vi "WidthEstimation.vi"(2 "maximum index":i32[](array[numeric]), 3 "maximium":dbl, 4 "2D Gaussian Data":dbl[][](array[numeric])) -> (0 "wy Estimated":dbl, 1 "wx Estimated":dbl)   [LabVIEW 2015]
panel:
  out "wx left":i32
  out "value wx left":dbl
  out "wx right":i32
  out "value wx right":dbl
  out "wy up":i32
  out "value wy up":dbl
  out "wy down":i32
  out "value wy down":dbl
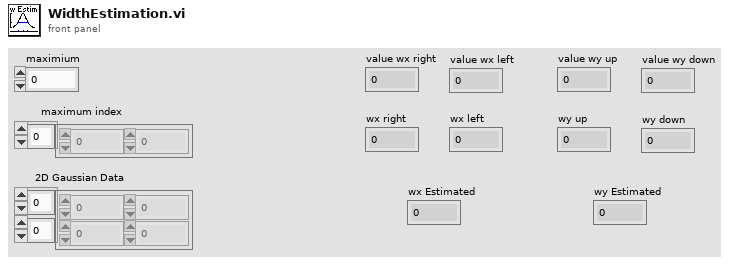
[diagram p1: front panel]
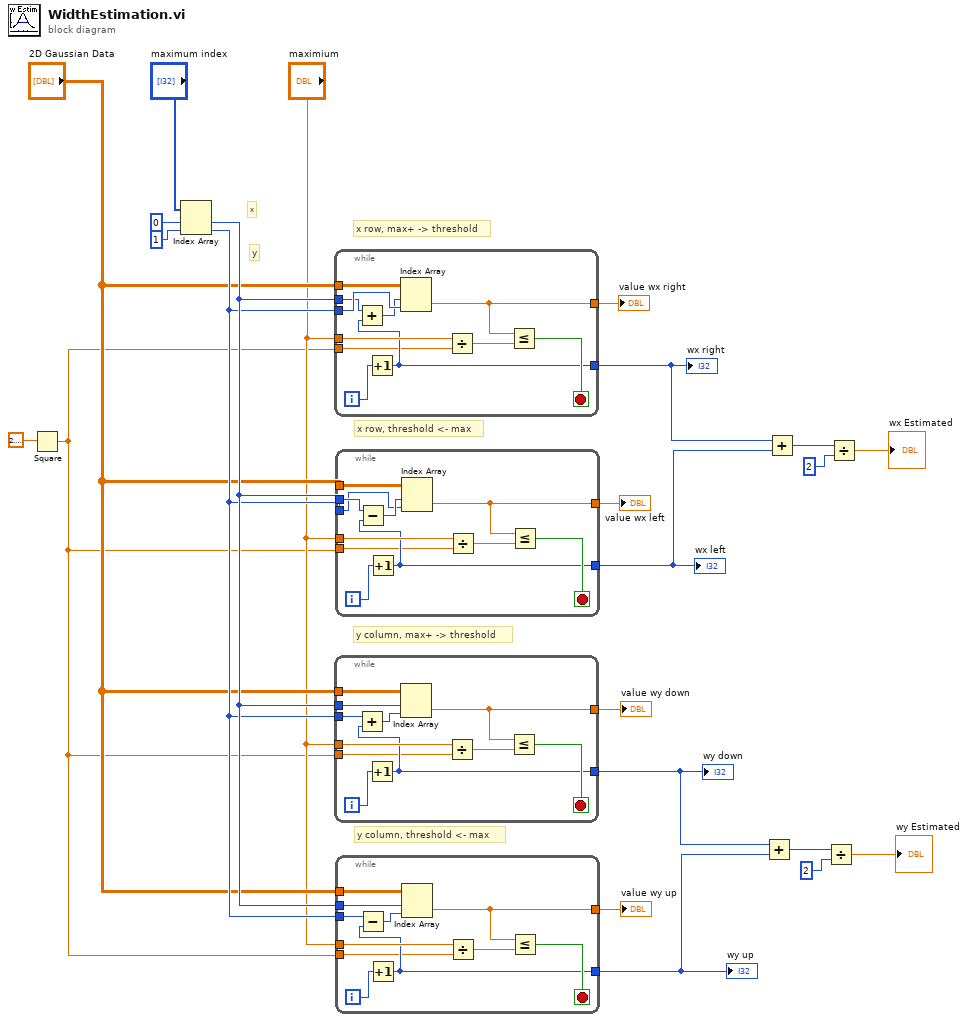
[diagram p0: block diagram]
diagram:
  # "x row, threshold <- max"
  # "x row, max+ -> threshold"
  # "y column, threshold <- max"
  # "y column, max+ -> threshold"
  # "y"
  # "x"
  n1 = Square(x=2.718281828459045) -> (x^2=w1:dbl)
  n2 = Index Array(array="maximum index", index #1=0 ("index"), index #2=1 ("index")) -> (element #1=w13:i32, element #2=w12:i32)
  n3 = while {
    tunnel: "2D Gaussian Data" -> [w34]
    tunnel: w13 -> [w26]
    tunnel: w12 -> [w27]
    tunnel: [w30] -> w10
    tunnel: "maximium" -> [w31]
    tunnel: [w28] -> w14
    tunnel: w1 -> [w24]
    i -> [w29]
    stop <- w32 stop-if-true
    n4 = Increment(x=w29) -> (x+1=w28:i32)
    n5 = Add(x=w26, y=w28) -> (x+y=w25:i32)
    n6 = Index Array(array=w34, index (row)=w25, index (col)=w27) -> (element=w30:dbl)
    n7 = Divide(x=w31, y=w24) -> (x/y=w33:dbl)
    n8 = Less Or Equal?(x=w30, y=w33) -> (x <= y?=w32:bool)
  }
  "value wx right" <- w10
  "wx right" <- w14
  n9 = while {
    tunnel: "2D Gaussian Data" -> [w45]
    tunnel: w13 -> [w44]
    tunnel: w12 -> [w43]
    tunnel: [w38] -> w7
    tunnel: "maximium" -> [w39]
    tunnel: [w36] -> w20
    tunnel: w1 -> [w35]
    i -> [w37]
    stop <- w40 stop-if-true
    n10 = Increment(x=w37) -> (x+1=w36:i32)
    n11 = Add(x=w43, y=w36) -> (x+y=w42:i32)
    n12 = Index Array(array=w45, index (row)=w44, index (col)=w42) -> (element=w38:dbl)
    n13 = Divide(x=w39, y=w35) -> (x/y=w41:dbl)
    n14 = Less Or Equal?(x=w38, y=w41) -> (x <= y?=w40:bool)
  }
  "value wy down" <- w7
  "wy down" <- w20
  n15 = while {
    tunnel: "2D Gaussian Data" -> [w56]
    tunnel: w13 -> [w49]
    tunnel: w12 -> [w47]
    tunnel: [w52] -> w9
    tunnel: "maximium" -> [w53]
    tunnel: [w50] -> w15
    tunnel: w1 -> [w46]
    i -> [w51]
    stop <- w54 stop-if-true
    n16 = Increment(x=w51) -> (x+1=w50:i32)
    n17 = Subtract(x=w49, y=w50) -> (x-y=w48:i32)
    n18 = Index Array(array=w56, index (row)=w48, index (col)=w47) -> (element=w52:dbl)
    n19 = Divide(x=w53, y=w46) -> (x/y=w55:dbl)
    n20 = Less Or Equal?(x=w52, y=w55) -> (x <= y?=w54:bool)
  }
  "value wx left" <- w9
  "wx left" <- w15
  n21 = while {
    tunnel: "2D Gaussian Data" -> [w67]
    tunnel: w13 -> [w66]
    tunnel: w12 -> [w65]
    tunnel: [w60] -> w8
    tunnel: "maximium" -> [w61]
    tunnel: [w58] -> w21
    tunnel: w1 -> [w57]
    i -> [w59]
    stop <- w62 stop-if-true
    n22 = Increment(x=w59) -> (x+1=w58:i32)
    n23 = Subtract(x=w65, y=w58) -> (x-y=w64:i32)
    n24 = Index Array(array=w67, index (row)=w66, index (col)=w64) -> (element=w60:dbl)
    n25 = Divide(x=w61, y=w57) -> (x/y=w63:dbl)
    n26 = Less Or Equal?(x=w60, y=w63) -> (x <= y?=w62:bool)
  }
  "value wy up" <- w8
  "wy up" <- w21
  n27 = Add(x=w20, y=w21) -> (x+y=w18:i32)
  n28 = Add(x=w14, y=w15) -> (x+y=w16:i32)
  n29 = Divide(x=w18, y=2) -> (x/y=→"wy Estimated":dbl)
  n30 = Divide(x=w16, y=2) -> (x/y=→"wx Estimated":dbl)
